vi "ArduinoPlatinumThermometer.vi"() -> ()   [LabVIEW 2014]
uses:
  <vilib>/MakerHub/LINX/Public/Peripherals/Analog/Analog Read 1 Chan.vi
  <vilib>/MakerHub/LINX/Public/Peripherals/Analog/Analog Read N Chans.vi
  <vilib>/MakerHub/LINX/Private/Local IO/LinxAnalogRead.vi
  <vilib>/MakerHub/LINX/Public/Utilities/Check Channel.vi
  <vilib>/MakerHub/LINX/Public/Utilities/Open Serial.vi
  <vilib>/MakerHub/LINX/Private/Utilties/Generate Error.vi
  <vilib>/MakerHub/LINX/LMH-LINX.lvlib
panel:
  out "Resistance":dbl format="%#_4f"
  out "Temperature":dbl format="%#_3g"
  out "Temperature":dbl(graph)
  out "Total V":dbl format="%#_2g"
  in  "VISA resource name":refnum<visa-resource-name>="COM5"
  in  "stop":bool
  out "Therm V":dbl format="%#_3g"
  out "Device Name":string
  out "Error In":errorcluster
  out "Error Out":errorcluster={"status"=FALSE, "code"=1073676294, "source"="VISA Read in LVH-LINX.lvlib:Device.lvlib:Serial Read.vi->LVH-LINX.lvlib:Device.lvlib:Wait For Packet.vi->LVH-LINX.lvlib:Device.lvlib:Send Command.vi->LVH-LINX.lvlib:Device.lvlib:Get DIO Channels.vi->LVH-LINX.lvlib:Device.lvlib:Load Device Config.vi->LVH-LINX.lvlib:Device.lvlib:Initialize Device.vi->LVH-LINX.lvlib:Initialize.vi->Untitled 2"}
  in  "Baud Rate":T1(ring)
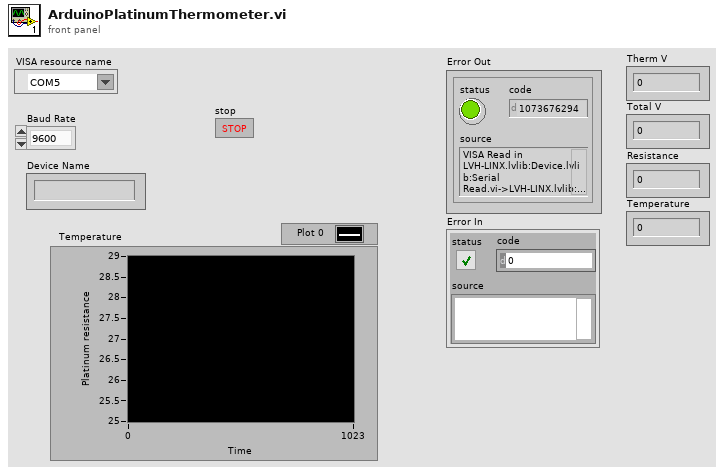
[diagram p1: front panel]
types:
  T1 = enum16{"9600", "14400", "19200", "28800", "38400", "57600", "115200"}
  T2 = typedef "LMH-LINX.lvlib/LINX Ref.ctl" = cluster{"IO":T3, "Interface":T4, "LINX Device Config":T5}
  T3 = typedef "LMH-LINX.lvlib/Platform.ctl" = enum16{"Remote", "Local"}
  T4 = typedef "LMH-LINX.lvlib/Interface.ctl" = enum16{"Serial", "TCP"}
  T5 = typedef "LMH-LINX.lvlib/Device.lvlib/LINX Device Config.ctl" = cluster{"Interface":T4, "COM Port":refnum<visa-resource-name>, "TCP Configuration":T6, "Device Family":u8, "Device ID":u8, "Device Name":string, "TCP Ref":refnum<k5>, "Channels":T7}
  T6 = typedef "LMH-LINX.lvlib/Device.lvlib/TCP Config.ctl" = cluster{"IP Address":string, "Port":u16}
  T7 = typedef "LMH-LINX.lvlib/Channels.ctl" = cluster{"DI":u8[], "DO":u8[], "AI":u8[], "AO":u8[], "PWM":u8[], "QE":u8[], "UART":u8[], "I2C 2":u8[], "SPI":u8[], "CAN":u8[], "Servo":u8[], "AI Ref (V)":dbl, "AI Resolution (Bits)":u8, "AO Ref (V)":dbl, "AO Resolution (Bits)":u8}
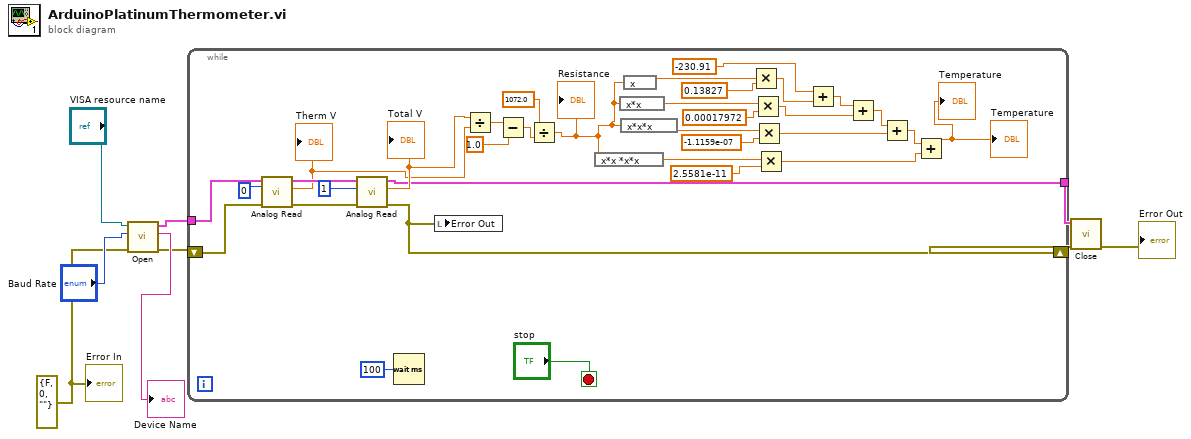
[diagram p0: block diagram]
diagram:
  w2 = errorcluster {"status"=FALSE, "code"=0, "source"=""} ("Error In")
  n1 = call-poly <vilib>:"Open.vi"("Error In"=w2, "Baud Rate Override"="Baud Rate", "Serial Port"="VISA resource name") -> ("Error Out"=w3:errorcluster, "Device Name"=→"Device Name":string, "LINX Resource"=w6:T2)  [unwired: 6 in]
  n2 = while {
    tunnel: [w32] -> w9
    shift-right: [w35] -> w1
    shift-left: w3 -> [w40]
    tunnel: w6 -> [w41]
    stop <- "stop" stop-if-true
    n3 = call-poly <vilib>:"Analog Read.vi"("Error In"=w40, "Analog Channel"=u8 0, "LINX Resource"=w41) -> ("Error Out"=w36:errorcluster, "Voltage"=w33:dbl, "LINX Resource"=w38:T2)  [unwired: 5 in, 1 out]
    "Therm V" <- w33
    n4 = call-poly <vilib>:"Analog Read.vi"("Error In"=w36, "Analog Channel"=u8 1, "LINX Resource"=w38) -> ("Error Out"=w35:errorcluster, "Voltage"=w34:dbl, "LINX Resource"=w32:T2)  [unwired: 5 in, 1 out]
    "Total V" <- w34
    n5 = Wait (ms)(milliseconds to wait=u32 100) -> ()  [unwired: 1 out]
    n6 = local write "Error Out"(w35) -> ()
    n7 = Divide(x=w34, y=w33) -> (x/y=w31:dbl)
    n8 = Subtract(x=w31, y=1.0) -> (x-y=w28:dbl)
    n9 = Divide(x=1072.0 ("y"), y=w28) -> (x/y=w11:dbl)
    "Resistance" <- w11
    n10 = expression code="x*x *x*x"(w11) -> (w12:dbl)
    n11 = expression code="x*x"(w11) -> (w14:dbl)
    n12 = expression code="x*x*x"(w11) -> (w13:dbl)
    n13 = expression code="x"(w11) -> (w15:dbl)
    n14 = Multiply(x=w15, y=0.13827) -> (x*y=w22:dbl)
    n15 = Multiply(x=w14, y=0.00017972) -> (x*y=w20:dbl)
    n16 = Multiply(x=w13, y=-1.1159e-07) -> (x*y=w18:dbl)
    n17 = Multiply(x=w12, y=2.5581e-11) -> (x*y=w17:dbl)
    n18 = Add(x=-230.91, y=w22) -> (x+y=w21:dbl)
    n19 = Add(x=w21, y=w20) -> (x+y=w19:dbl)
    n20 = Add(x=w19, y=w18) -> (x+y=w16:dbl)
    n21 = Add(x=w16, y=w17) -> (x+y=→"Temperature" →"Temperature":dbl)
  }
  n22 = call <vilib>:"Close.vi"("Error In"=w1, "LINX Resource"=w9) -> ("Error Out"=→"Error Out":errorcluster)  [unwired: 9 in]
  "Error In" <- w2
